vi "serial open.vi"() -> ()   [LabVIEW 2020]
panel:
  in  "duplicate session (F)":bool
  in  "access mode":u32
  out "error out":errorcluster
  in  "VISA resource name":refnum<visa-resource-name>
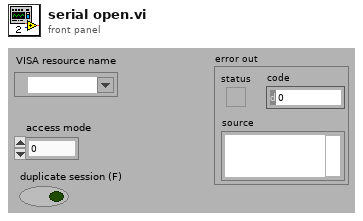
[diagram p1: front panel]
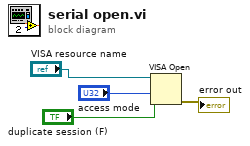
[diagram p0: block diagram]
diagram:
  n1 = VISA Open(duplicate session (F)="duplicate session (F)", access mode="access mode", VISA resource name="VISA resource name") -> (error out=→"error out":errorcluster)  [unwired: 2 in, 1 out]
